vi "Find Average and Std Dev.vi"(5 "ROI":u8[][](array[numeric]), 7 "Use ROI?":bool, 11 "Depth History":refnum<queue>) -> (1 "Std Dev.":dbl, 3 "Average Depth":dbl, 4 "Filtered Depth Values":dbl[](array[numeric]))   [LabVIEW 2018]
uses:
  <vilib>/Analysis/NI_AALBase.lvlib
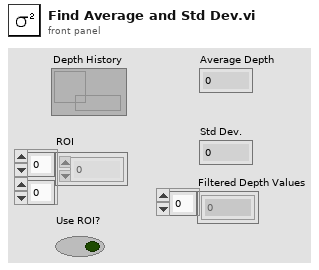
[diagram p1: front panel]
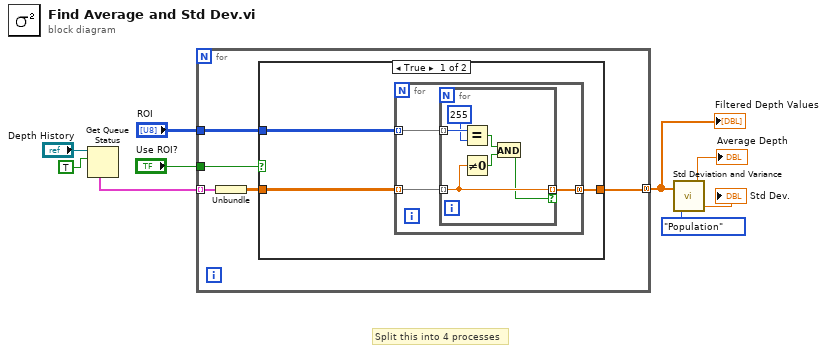
[diagram p0: block diagram]
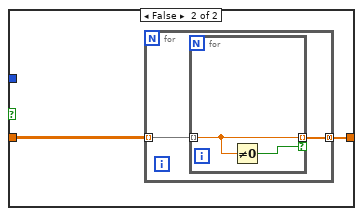
[diagram p2: hidden frame]
diagram:
  # "Split this into 4 processes"
  n1 = Get Queue Status(queue="Depth History", return elements? (F)=TRUE) -> (elements=w7:cluster{dbl[][]}[])  [unwired: 1 in, 7 out]
  n2 = for {
    tunnel: w7 -> [w14] mode=indexing
    tunnel: [w12] -> w3 mode=concatenating
    tunnel: "ROI" -> [w11]
    tunnel: "Use ROI?" -> [w10]
    n3 = Unbundle(w14) -> (w13:dbl[][])
    n4 = case shown="True" w10 {
      tunnel: w13 -> [w17 w28]
      tunnel: [w16 w27] -> w12
      tunnel: w11 -> [w15 _]
      frame True {
        n5 = for {
          tunnel: w17 -> [w20] mode=indexing
          tunnel: [w19] -> w16 mode=concatenating
          tunnel: w15 -> [w18] mode=indexing
          n6 = for {
            tunnel: w20 -> [w24] mode=indexing
            tunnel: [w24] -> w19 mode=indexing if=w21
            tunnel: w18 -> [w26] mode=indexing
            n7 = Equal?(x=w26, y=u8 255) -> (x = y?=w22:bool)
            n8 = Not Equal To 0?(x=w24) -> (x != 0?=w23:bool)
            n9 = And(x=w22, y=w23) -> (x .and. y?=w21:bool)
          }
        }
      }
      frame False {
        n10 = for {
          tunnel: w28 -> [w30] mode=indexing
          tunnel: [w29] -> w27 mode=concatenating
          n11 = for {
            tunnel: w30 -> [w32] mode=indexing
            tunnel: [w32] -> w29 mode=indexing if=w31
            n12 = Not Equal To 0?(x=w32) -> (x != 0?=w31:bool)
          }
        }
      }
    }
  }
  "Filtered Depth Values" <- w3
  n13 = call <vilib>:"Std Deviation and Variance.vi"("X"=w3, "Weighting (Sample)"=enum16{"Sample", "Population"}."Population") -> ("mean"=→"Average Depth":dbl, "variance"=→"Std Dev.":dbl)  [unwired: 1 out]
